vi "Read Stream.lvclass.vi"(8 "error in (no error)":errorcluster, 11 "Client in":refnum<class "Client.lvclass">) -> (0 "error out":errorcluster, 2 "Stream.lvclass":refnum<class "Stream.lvclass">, 3 "Client out":refnum<class "Client.lvclass">)   [LabVIEW 2018, in "Client.lvclass"]
uses:
  Client.lvclass
  Comm/Stream/Stream.lvclass
  Client.lvclass/Client.ctl
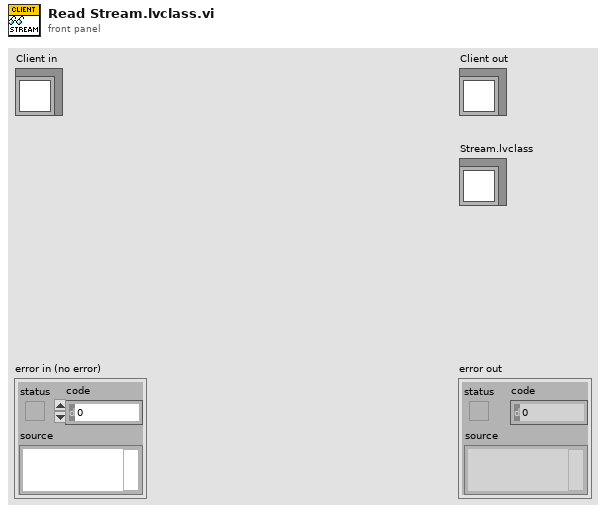
[diagram p1: front panel]
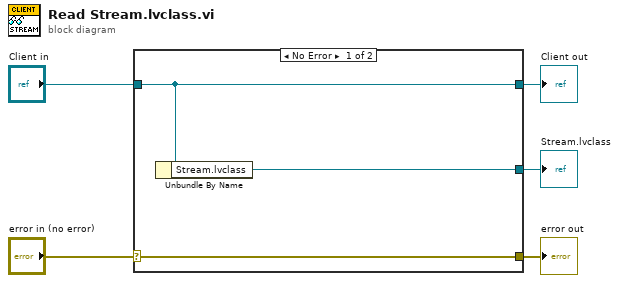
[diagram p0: block diagram]
diagram:
  n1 = case shown="No Error" "error in (no error)" {
    selector: "error in (no error)" -> [w8 w9]
    tunnel: [w8 w9] -> w4
    tunnel: [w7 w10] -> w2
    tunnel: "Client in" -> [w7 w10]
    tunnel: [w6 _] -> w1
    frame No Error {
      n2 = Unbundle By Name(w7) -> ("Stream.lvclass"=w6:refnum<class "Stream.lvclass">)
    }
    frame Error {
    }
  }
  "error out" <- w4
  "Client out" <- w2
  "Stream.lvclass" <- w1
